vi "Bark Url Encode.vi"(8 "Message":string, 9 "Title":string, 10 "Group":string, 11 "Url":string) -> (3 "UrlEncode":string)   [LabVIEW 2016, in "Bark.lvlib" / "Bark.lvclass"]
uses:
  Bark.lvclass
  System.Web
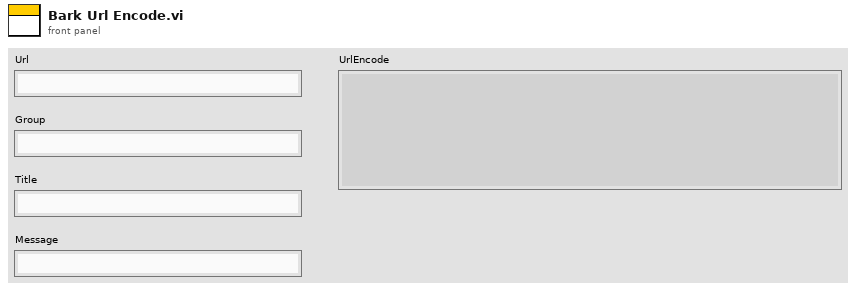
[diagram p1: front panel]
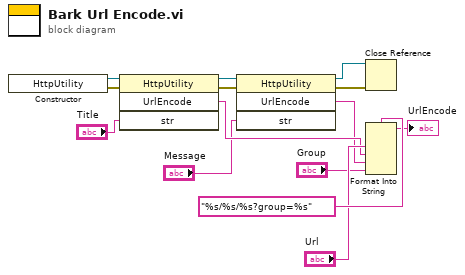
[diagram p0: block diagram]
diagram:
  n1 = constructor class="HttpUtility"() -> (reference out=w12:refnum<k24>, error out=w11:errorcluster)  [unwired: 3 in, 1 out]
  n2 = invoke class="HttpUtility" method="UrlEncode"(reference=w12, error in=w11, "str"="Title") -> (reference out=w7:refnum<k24>, error out=w6:errorcluster, "UrlEncode"=w8:string)  [unwired: 1 in, 1 out]
  n3 = invoke class="HttpUtility" method="UrlEncode"(reference=w7, error in=w6, "str"="Message") -> (reference out=w5:refnum<k24>, error out=w4:errorcluster, "UrlEncode"=w2:string)  [unwired: 1 in, 1 out]
  n4 = Close Reference(reference=w5, error in (no error)=w4) -> ()  [unwired: 1 out]
  n5 = Format Into String(format string="%s/%s/%s?group=%s" ("格式字符串"), "Url", w8, w2, "Group") -> (resulting string=→"UrlEncode":string)  [unwired: 2 in, 1 out]
